vi "Remove Module from Project.vi"(6 "TreeControl in":refnum<vi>, 8 "error in":errorcluster, 11 "Data Cluster In":T1={"Project"=refnum, "Current Selection"={"Library"=refnum, "VI"=refnum}, "Module ID"=-1, "Tree Selection"=""}) -> (0 "error out":errorcluster, 3 "Data Cluster Out":T1={"Project"=refnum, "Current Selection"={"Library"=refnum, "VI"=refnum}, "Module ID"=-1, "Tree Selection"=""})   [LabVIEW 2020, in "Panther Dashboard.lvlib"]
doc: "Gets the Singleton and Cloneable references and creates a list of each type of DQMH Modules"
uses:
  Panther Dashboard.lvlib
  Module Data--cluster.ctl
  Class/Project/Project.lvclass
  C:/GitClones/PantherDashboard/src/LabVIEW/Panther Dashboard/Class/LabVIEWItem/LabVIEWItem.lvclass
  Class/Library/Library.lvclass
  Class/VI/VI.lvclass
  Class/Project/Project.lvclass/Project.ctl
  Class/LabVIEWItem/LabVIEWItem.lvclass/LabVIEWItem.ctl
  Class/Library/Library.lvclass/Library.ctl
  Class/LabVIEWItem/Read Item Tag.vi
  Class/Project/Read Libraries.vi
  Class/Library/Read Library Ref.vi
  Class/LabVIEWItem/Read Item Name.vi
  Class/Project/Write Libraries.vi
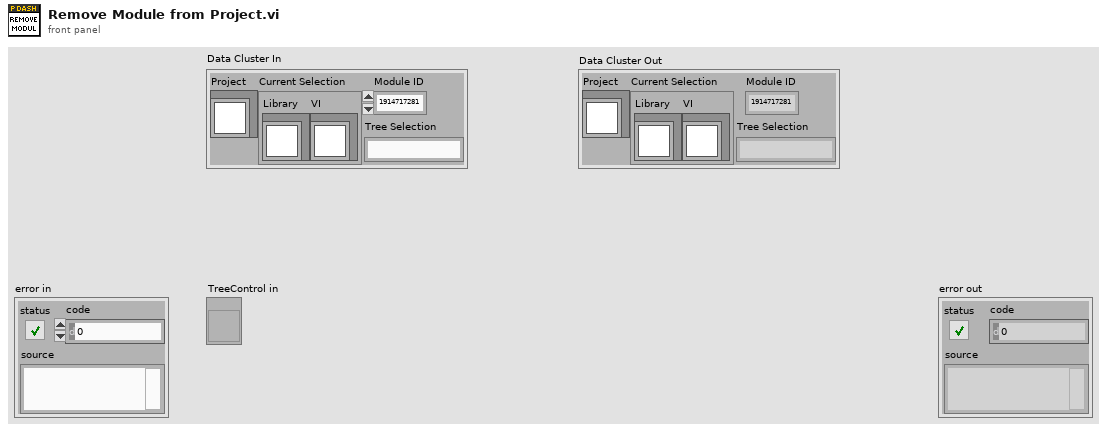
[diagram p1: front panel]
types:
  T1 = typedef "Panther Dashboard.lvlib/Module Data--cluster.ctl" = cluster{"Project":refnum<class "Project.lvclass">, "Current Selection":cluster{"Library":refnum<class "Library.lvclass">, "VI":refnum<class "VI.lvclass">}, "Module ID":i32, "Tree Selection":string}
  T2 = typedef "Tree Map.lvlib/Tree Map Data.ctl" = map{string, cluster{"Child Paths Set":set{string}, "Name":string, "Data":string, "Attributes":map{string, string}}}
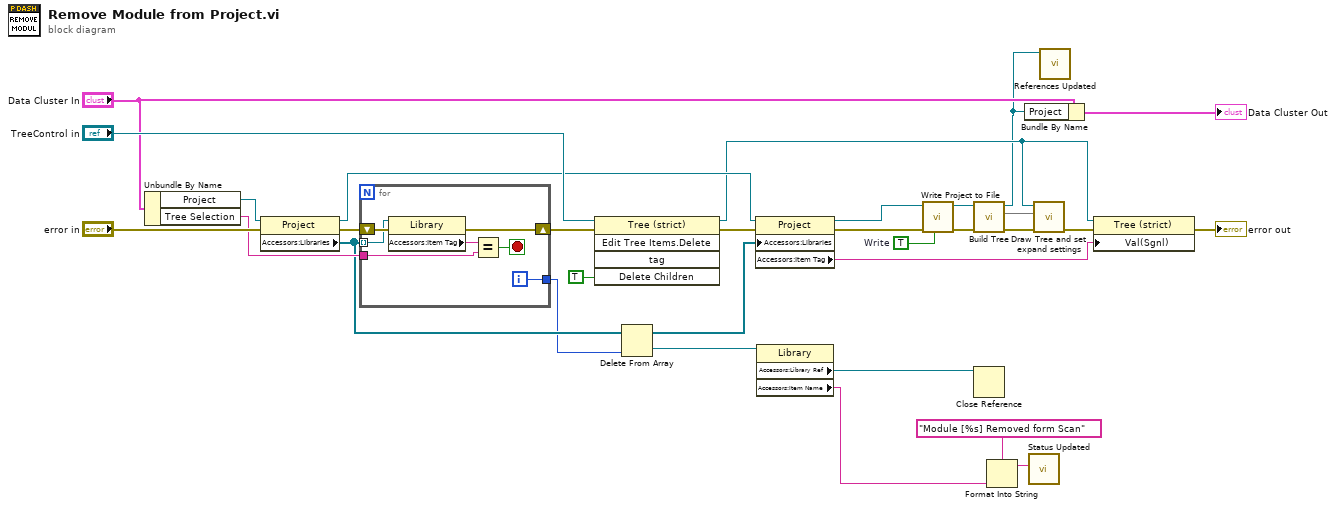
[diagram p0: block diagram]
diagram:
  w21 = TRUE  # Write
  n1 = Unbundle By Name("Data Cluster In") -> ("Project"=w16:refnum<class "Project.lvclass">, "Tree Selection"=w15:string)
  n2 = property class="Project"(reference=w16, error in="error in") -> (reference out=w11:refnum<class "Project.lvclass">, error out=w31:errorcluster, "Accessors:Libraries"=w14:refnum<class "Library.lvclass">[])
  n3 = for {
    tunnel: w14 -> [w36] mode=indexing
    tunnel: w15 -> [w34]
    tunnel: [w32] -> w4
    shift-right: [w37] -> w29
    shift-left: w31 -> [w38]
    i -> [w32]
    stop <- w33 stop-if-true
    n4 = property class="Library"(reference=w36, error in=w38) -> (error out=w37:errorcluster, "Accessors:Item Tag"=w35:string)  [unwired: 1 out]
    n5 = Equal?(x=w35, y=w34) -> (x = y?=w33:bool)
  }
  n6 = invoke class="Tree (strict)" method="Edit Tree Items.Delete"(reference="TreeControl in", error in=w29, "Delete Children"=TRUE ("Delete Children?")) -> (reference out=w9:refnum<vi>, error out=w28:errorcluster)  [unwired: 2 in, 3 out]
  n7 = Delete From Array "Delete From Array"(array=w14, index=w4) -> (deleted portion=w3:refnum<class "Library.lvclass">, array with subset deleted=w13:refnum<class "Library.lvclass">[])  [unwired: 1 in]
  n8 = property class="Project"(reference=w11, error in=w28, "Accessors:Libraries"=w13) -> (reference out=w7:refnum<class "Project.lvclass">, error out=w25:errorcluster, "Accessors:Item Tag"=w1:string)
  n9 = property class="Library"(reference=w3) -> ("Accessors:Library Ref"=w12:refnum<vi>, "Accessors:Item Name"=w5:string)  [unwired: 1 in, 2 out]
  n10 = call "Write Project to File.vi"("Write"=w21, "error in"=w25, "Project In"=w7) -> ("error out"=w24:errorcluster, "Project Out"=w6:refnum<class "Project.lvclass">)  [unwired: 6 in, 1 out]
  n11 = call "Build Tree.vi"("error in"=w24, "Project in"=w6) -> ("error out"=w27:errorcluster, "Tree Map Out"=w10:T2, "Project Out"=w8:refnum<class "Project.lvclass">)  [unwired: 7 in]
  n12 = Close Reference(reference=w12) -> ()  [unwired: 1 in, 1 out]
  n13 = Format Into String(format string="Module [%s] Removed form Scan" ("Status"), w5) -> (resulting string=w19:string)  [unwired: 2 in, 1 out]
  n14 = Bundle By Name(cluster="Data Cluster In", "Project"=w8) -> (→"Data Cluster Out":T1)
  n15 = call "Status Updated.vi"("Status"=w19) -> ()  [unwired: 10 in, 1 out]
  n16 = call "Draw Tree and set expand settings.vi"("error in"=w27, "Tree Map In"=w10, "TreeControl in"=w9) -> ("error out"=w2:errorcluster)  [unwired: 8 in]
  n17 = call "References Updated.vi"("Project"=w8) -> ()  [unwired: 10 in, 1 out]
  n18 = property class="Tree (strict)"(reference=w9, error in=w2, "Val(Sgnl)"=w1) -> (error out=→"error out":errorcluster)  [unwired: 1 out]
